vi "Get Class Path.vi"(0 "Device in":refnum<class "Device.lvclass">, 11 "Error in":errorcluster) -> (4 "Device out":refnum<class "Device.lvclass">, 6 "Class Path":path, 15 "Error out":errorcluster)   [LabVIEW 2020, in "Device.lvclass"]
doc: "Get the file path for the input class object"
uses:
  Device.lvclass
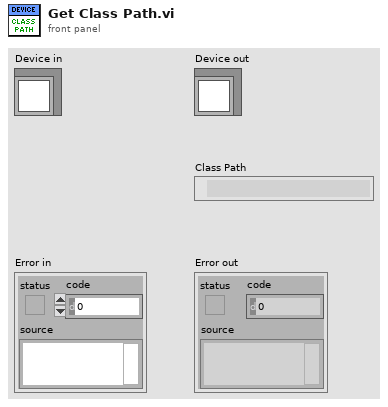
[diagram p1: front panel]
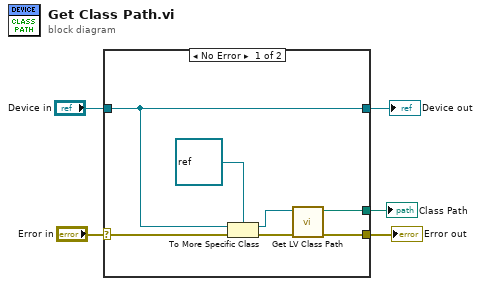
[diagram p0: block diagram]
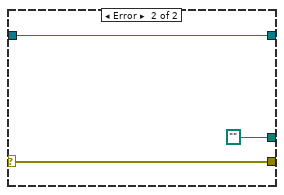
[diagram p2: hidden frame]
diagram:
  n1 = case shown="No Error" "Error in" {
    selector: "Error in" -> [w10 w15]
    tunnel: [w12 w15] -> w4
    tunnel: [w8 w14] -> w2
    tunnel: "Device in" -> [w8 w14]
    tunnel: [w11 path ""] -> w1
    frame No Error {
      n2 = To More Specific Class(target class=refnum<class> refnum ("LabVIEW Object"), reference=w8, error in=w10) -> (specific class reference=w7:refnum<class>, error out=w9:errorcluster)
      n3 = call <vilib>:"Get LV Class Path.vi"("error in (no error)"=w9, "object"=w7) -> ("error out"=w12:errorcluster, "class path"=w11:path)  [unwired: 8 in]
    }
    frame Error {
    }
  }
  "Error out" <- w4
  "Device out" <- w2
  "Class Path" <- w1
